vi "Get Matrix Data.vi"(6 "Index":i32, 7 "2D Plotmatrix Datatype.lvclass in":refnum<class "XY Plot Matrix Datatype.lvclass">, 8 "error in (no error)":errorcluster, 10 "Matrix Representation Array In":T1) -> (0 "error out":errorcluster, 2 "Matrix Representation Array Out":T1, 5 "2D Plotmatrix Datatype.lvclass out":refnum<class "XY Plot Matrix Datatype.lvclass">)   [LabVIEW 2020, in "XY Plot Matrix Datatype.lvclass"]
uses:
  <vilib>/Math Plots/2D Math Plots/XY Plot Matrix/XY Plot Matrix Datatype/XY Plot Matrix Datatype.lvclass
  <vilib>/Math Plots/2D Math Plots/XY Plot Matrix/XY Plot Matrix/Typedef/Mulitmatrix Representation.ctl
  <vilib>/Math Plots/2D Math Plots/XY Plot Matrix/XY Plot Matrix/Typedef/Matrix Representation.ctl
  <vilib>/Math Plots/2D Math Plots/2D Plot/2D Plot/Typedef/Range Cluster.ctl
  <vilib>/Math Plots/2D Math Plots/XY Plot Matrix/XY Plot Matrix/XY Plot Matrix.lvclass
  <vilib>/Math Plots/2D Math Plots/2D Plot/2D Plot/2D Plot.lvclass
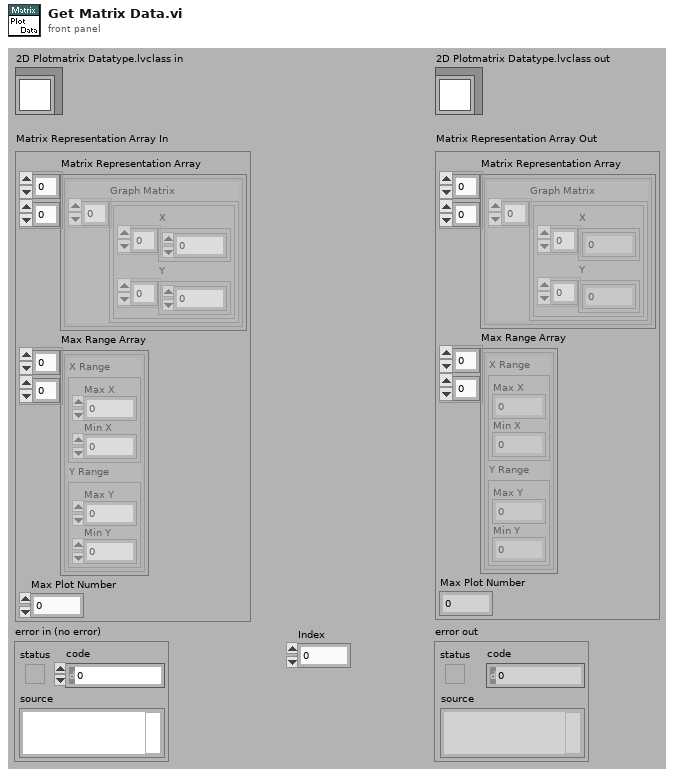
[diagram p1: front panel]
types:
  T1 = typedef "XY Plot Matrix.lvclass/Mulitmatrix Representation.ctl" = cluster{"Matrix Representation Array":T2[][], "Max Range Array":T3[][], "Max Plot Number":i32}
  T2 = typedef "XY Plot Matrix.lvclass/Matrix Representation.ctl" = cluster{"Graph Matrix":cluster{"X":dbl[], "Y":dbl[]}[]}
  T3 = typedef "2D Plot.lvclass/Range Cluster.ctl" = cluster{"X Range":cluster{"Max X":dbl, "Min X":dbl}, "Y Range":cluster{"Max Y":dbl, "Min Y":dbl}}
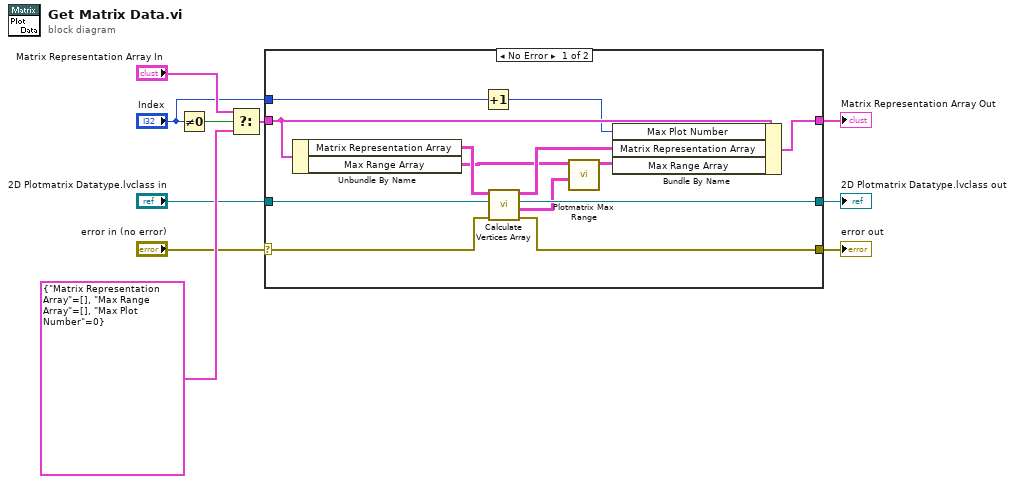
[diagram p0: block diagram]
diagram:
  n1 = Not Equal To 0?(x="Index") -> (x != 0?=w9:bool)
  n2 = Select(t="Matrix Representation Array In", s=w9, f=T1 {"Matrix Representation Array"=[], "Max Range Array"=[], "Max Plot Number"=0} ("Multiplot Representation In")) -> (s? t:f=w5:T1)
  n3 = case shown="No Error" "error in (no error)" {
    selector: "error in (no error)" -> [w19 w24]
    tunnel: "2D Plotmatrix Datatype.lvclass in" -> [w20 w25]
    tunnel: w5 -> [w23 w26]
    tunnel: [w18 w24] -> w4
    tunnel: [w22 w26] -> w3
    tunnel: [w21 w25] -> w2
    tunnel: "Index" -> [w15 _]
    frame No Error {
      n4 = Unbundle By Name(w23) -> ("Matrix Representation Array"=w17:T2[][], "Max Range Array"=w13:T3[][])
      n5 = Increment(x=w15) -> (x+1=w11:i32)
      n6 = call <vilib>:"Calculate Vertices Array.vi"("error in (no error)"=w19, "2D Plotmatrix Datatype.lvclass in"=w20, "Matrix Representation Array"=w17) -> ("error out"=w18:errorcluster, "Max Range Array"=w14:T3[][], "2D Plotmatrix Datatype.lvclass out"=w21:refnum<class "XY Plot Matrix Datatype.lvclass">, "Matrix Representation Array"=w16:T2[][])  [unwired: 5 out]
      n7 = call <vilib>:"Plotmatrix Max Range.vi"("Current Range Array"=w14, "Max Range Array In"=w13) -> ("Max Range Array Out"=w12:T3[][])  [unwired: 9 out]
      n8 = Bundle By Name(cluster=w23, "Max Plot Number"=w11, "Matrix Representation Array"=w16, "Max Range Array"=w12) -> (w22:T1)
    }
    frame Error {
    }
  }
  "2D Plotmatrix Datatype.lvclass out" <- w2
  "error out" <- w4
  "Matrix Representation Array Out" <- w3
